vi "Set SPI Transfer Length 128-bit.vi"(8 "error in":errorcluster, 9 "Set? (T)":bool=TRUE, 10 "Transfer Length (bits)":u8=4 min=4, 11 "SPI Engine Resources":T1={"To SPI Engine Data FIFO"="DLU To SPI Engine Data FIFO", "From SPI Engine Data FIFO"="SPI Engine to DLU Data FIFO", "Data to SPI Engine Cache Register"="Data to SPI Engine (Cache)", "SPI Transaction Settings Cache Register"="SPI PHY Settings to SPI Engine (Cache)"}) -> (0 "error out":errorcluster, 3 "SPI Engine Resources":T1={"To SPI Engine Data FIFO"="DLU To SPI Engine Data FIFO", "From SPI Engine Data FIFO"="SPI Engine to DLU Data FIFO", "Data to SPI Engine Cache Register"="Data to SPI Engine (Cache)", "SPI Transaction Settings Cache Register"="SPI PHY Settings to SPI Engine (Cache)"})   [LabVIEW 2015, in "SPI API.lvlib"]
doc: "This VI sets the transfer length in bits for a transaction by the SPI Engine. The transfer length corresponds to the number of bits to be transmitted by the SPI Engine on the MOSI line, as well as the number of bits to be read by the SPI Engine on the MISO line."
uses:
  Controls/SPI Engine Resources 128-bit.ctl
  <vilib>/rvi/DataTransferAndStorage/Container/Common/niFpgaContainerExecOnDevCompGetState.vi
  <vilib>/rvi/Emulation/niFpgaEmulationIsFPGAContextNoSignature.vi
  <vilib>/rvi/DataTransferAndStorage/Container/Common/niFpgaContainerGetUniqueNameForEmu.vi
  <vilib>/rvi/Memory/Memory_Emulation/niFpgaMemoryEmulationCacheClearOnFirstRun.vi
  <vilib>/rvi/Memory/Memory_Emulation/nirvimemoryEmulationManagerCache_MakeExclusive.vi
  <vilib>/rvi/Memory/Memory_Emulation/niFpgaMemoryEmulationValidateCache.vi
  <vilib>/rvi/Memory/Memory_Emulation/nirvimemoryEmulationManagerCache_InsertValue.vi
  <vilib>/Utility/error.llb/Clear Errors.vi
  <vilib>/rvi/Memory/Memory_Emulation/nirvimemoryEmulationManagerCache_ReleaseExclusive.vi
  <vilib>/rvi/Memory/Memory_Emulation/nirvimemoryEmulationManagerCache_GetValue.vi
  <vilib>/rvi/Memory/Memory_Emulation/nirvimemoryEmulationManagerCache_SetValue.vi
  <vilib>/rvi/Emulation/niFpgaProcessEmulError.vi
  <vilib>/rvi/Emulation/niFpgaSctlEmulationGetInTimedLoop.vi
  <vilib>/rvi/DataTransferAndStorage/Container/XNode/niFpgaContainer.xnode
  <vilib>/rvi/DataTransferAndStorage/Register/Emulation/niFpgaRegisterEmulationRefIn.vi
  SPI API.lvlib
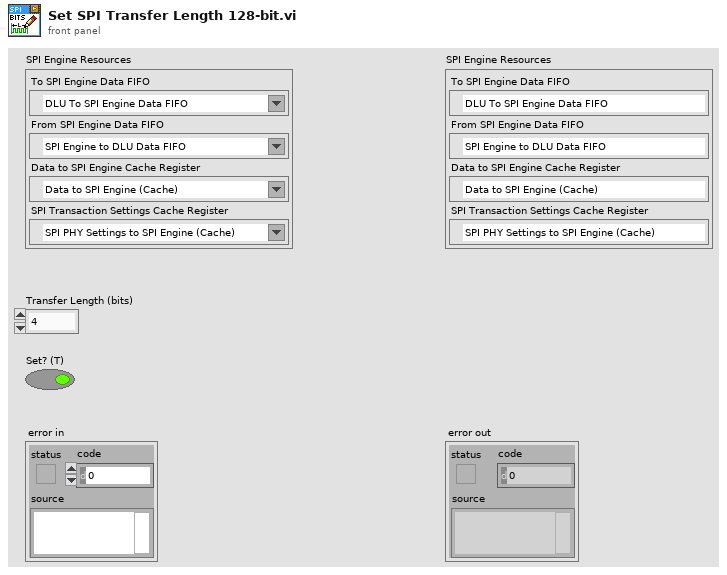
[diagram p1: front panel]
types:
  T1 = typedef "SPI API.lvlib/SPI Engine Resources 128-bit.ctl" = cluster{"To SPI Engine Data FIFO":refnum<k21>, "From SPI Engine Data FIFO":refnum<k21>, "Data to SPI Engine Cache Register":refnum<k21>, "SPI Transaction Settings Cache Register":refnum<k21>}
  T2 = cluster{"Chip Select ID":u8, "SPI Physical Settings":cluster{"Divide Value":u8, "Transfer Length (bits)":u8, "CS Asserted Polarity":bool, "Clock Polarity (CPOL)":bool, "Clock Phase (CPHA)":bool, "Lengthen MISO Setup":bool, "Direction Change Bit":u8, "MOSI Starts as Output":bool, "Tristatable MOSI":bool}}
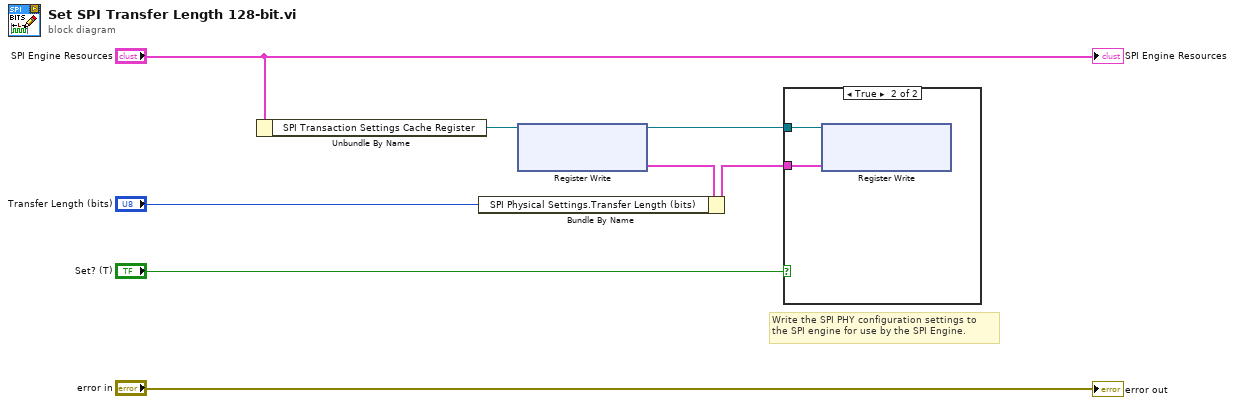
[diagram p0: block diagram]
diagram:
  # "Write the SPI PHY configuration settings to\nthe SPI engine for use by the SPI Engine."
  n1 = Unbundle By Name("SPI Engine Resources") -> ("SPI Transaction Settings Cache Register"=w6:refnum<k21>)
  n2 = xnode ("Register Write")("Register In"=w6) -> ("Data"=w2:T2, "Register Out"=w5:refnum<k21>)
  n3 = Bundle By Name(cluster=w2, "SPI Physical Settings.Transfer Length (bits)"="Transfer Length (bits)") -> (w3:T2)
  n4 = case shown="True" "Set? (T)" {
    tunnel: w5 -> [_ w10]
    tunnel: w3 -> [_ w9]
    frame False {
    }
    frame True {
      n5 = xnode ("Register Write")("Data"=w9, "Register In"=w10) -> ()  [unwired: 1 out]
    }
  }
  "error out" <- "error in"
  "SPI Engine Resources" <- "SPI Engine Resources"
